vi "DestroyBroadcastEvents.vi"(8 "error in (no error)":errorcluster) -> (0 "error out":errorcluster)   [LabVIEW 2018, in "SyncModule.lvlib"]
uses:
  SyncModule.lvlib
  SyncBroadcastEvents.ctl
  clEventType.ctl
panel:
  out "clBroadcastEvents":T1
  # "If you want to add other Broadcast Events, open this typedef, copy an existing event and rename it to your event name.\n\nNext create an \"arg\" typedef for the  data and put it into PublicAPI/Arguments/Broadcasts\n\nAfter that, you will need to create a new roadcast vi in Protected/Broadcast.  Look at DidInit.vi or the reportError.vi as examples."
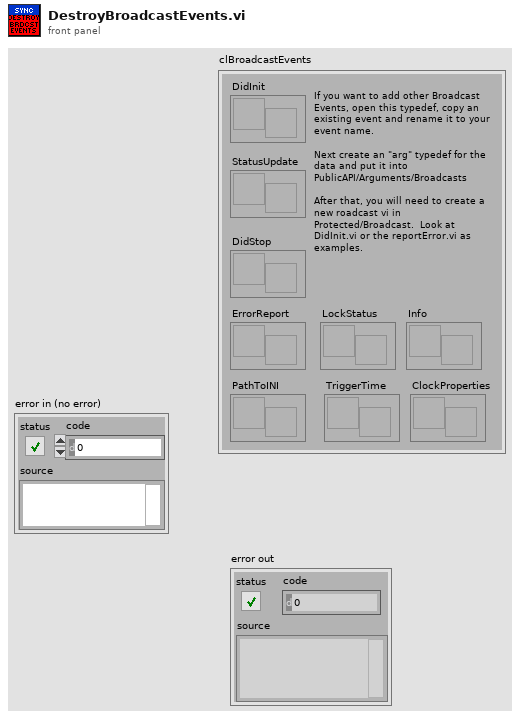
[diagram p1: front panel]
types:
  T1 = typedef "SyncModule.lvlib/SyncBroadcastEvents.ctl" = cluster{"DidInit":refnum<user-event>, "StatusUpdate":refnum<user-event>, "ErrorReport":refnum<user-event>, "DidStop":refnum<user-event>, "PathToINI":refnum<user-event>, "TriggerTime":refnum<user-event>, "LockStatus":refnum<user-event>, "Info":refnum<user-event>, "ClockProperties":refnum<user-event>}
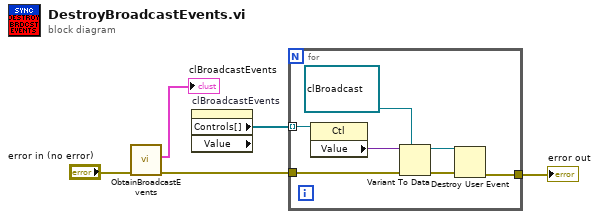
[diagram p0: block diagram]
diagram:
  n1 = call "ObtainBroadcastEvents.vi"("error in (no error)"="error in (no error)") -> ("error out"=w2:errorcluster, "SyncBroadcastEvents"=→"clBroadcastEvents":T1)  [unwired: 9 in]
  n2 = property on="clBroadcastEvents" class="Clust (strict)" props=["Controls[]", "Value"]() -> ("Controls[]"=w4:refnum<vi>[])  [unwired: 2 in, 3 out]
  n3 = for {
    tunnel: w4 -> [w12] mode=indexing
    tunnel: w2 -> [w9]
    tunnel: [w8] -> w5
    n4 = property class="Ctl"(reference=w12) -> ("Value"=w11:variant)  [unwired: 1 in, 2 out]
    n5 = Variant To Data(error in=w9, type=refnum<user-event> refnum ("DidInit"), Variant=w11) -> (data=w7:refnum<user-event>, error out=w10:errorcluster)
    n6 = Destroy User Event(user event=w7, error in=w10) -> (error out=w8:errorcluster)
  }
  "error out" <- w5
